vi "CallEngine.vi"(8 "error in (no error)":errorcluster, 10 "RT_Game.lvlib:Engine.lvclass":refnum<class "Engine.lvclass">, 11 "Game in":refnum<class "Game.lvclass">) -> (0 "error out":errorcluster, 2 "RT_Game.lvlib:Engine.lvclass 2":refnum<class "Engine.lvclass">, 3 "Game out":refnum<class "Game.lvclass">)   [LabVIEW 2019, in "RT_Game.lvlib" / "Game.lvclass"]
uses:
  Game.lvclass
  Engine/Engine.lvclass
  Engine/Engine.lvclass/Engine.ctl
  Engine/Write delta_t.vi
  Engine/Write Update_.vi
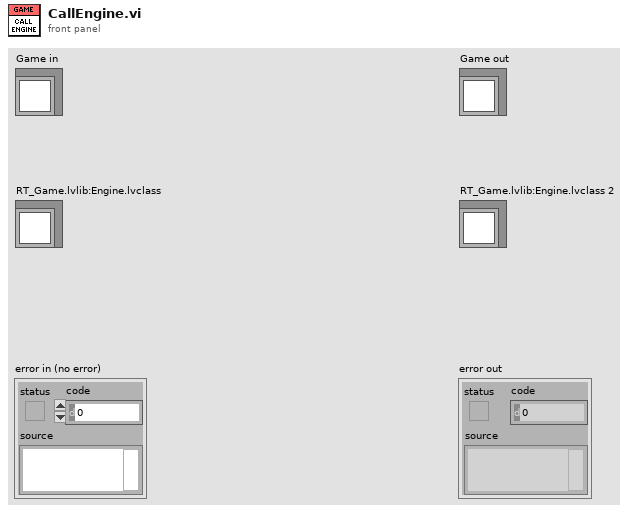
[diagram p1: front panel]
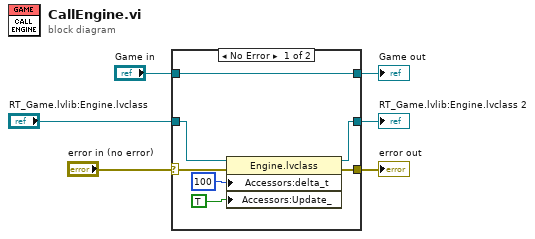
[diagram p0: block diagram]
diagram:
  n1 = case shown="No Error" "error in (no error)" {
    selector: "error in (no error)" -> [w12 w16]
    tunnel: [w11 w16] -> w5
    tunnel: [w13 w15] -> w3
    tunnel: "Game in" -> [w13 w15]
    tunnel: [w9 w14] -> w1
    tunnel: "RT_Game.lvlib:Engine.lvclass" -> [w10 w14]
    frame No Error {
      n2 = property class="Engine.lvclass"(reference=w10, error in=w12, "Accessors:delta_t"=u16 100 ("delta_t"), "Accessors:Update_"=TRUE ("Update_")) -> (reference out=w9:refnum<class "Engine.lvclass">, error out=w11:errorcluster)
    }
    frame Error {
    }
  }
  "error out" <- w5
  "Game out" <- w3
  "RT_Game.lvlib:Engine.lvclass 2" <- w1
